vi "Unit Test.vi"() -> ()   [LabVIEW 2018]
uses:
  LWS SLA-070/Distro/Projects/12170 Luminar LWS Base/Source/PPLs/Oscilloscope.lvlibp/Oscilloscope.lvclass
  PicoScope 3000a.lvclass
  C:/Projects/LWS SLA-070/Distro/Projects/12170 Luminar LWS Base/Source/PPLs/Oscilloscope.lvlibp/Oscilloscope.lvclass
  PicoScope 3000a.lvclass/PicoScope 3000a.ctl
  LWS SLA-070/Distro/Projects/12170 Luminar LWS Base/Source/PPLs/Oscilloscope.lvlibp/Custom Controls/Analog Channels.ctl
  LWS SLA-070/Distro/Projects/12170 Luminar LWS Base/Source/PPLs/Oscilloscope.lvlibp/Custom Controls/Volts per Division.ctl
  LWS SLA-070/Distro/Projects/12170 Luminar LWS Base/Source/PPLs/Oscilloscope.lvlibp
  ps3000a.dll
panel:
  out "Handle":i16
  in  "TimePicoSeconds":i32
  in  "Interleave":i16
  in  "Cycles":i16
  in  "ETS_Mode":i32
  out "Oscilloscope out":refnum<class "Oscilloscope.lvclass">
  out "Multiple Waveform":waveform(dbl)[](graph)
  in  "Waveform":enum16{"Single", "Multiple"}(ring)
  in  "Secs/div":dbl
  out "SingleWaveform":waveform(dbl)(graph)
  in  "Acquire":bool
  in  "Set Scale":bool
  in  "Stop":bool
  out "error out":errorcluster
  in  "error in (no error)":errorcluster
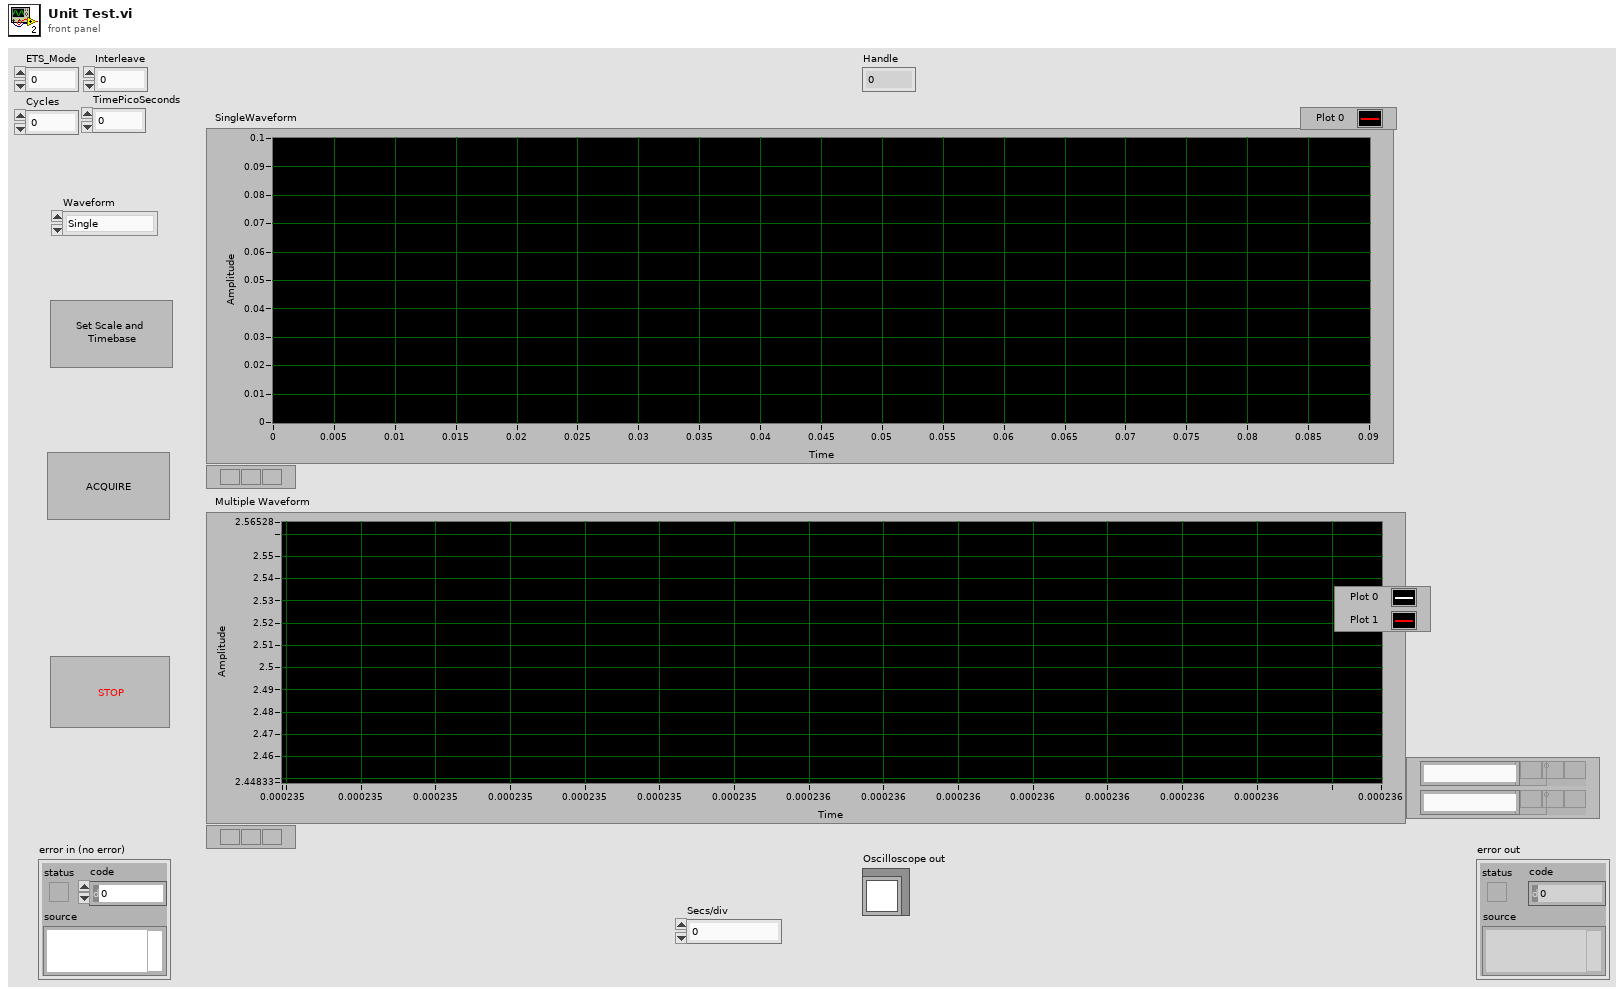
[diagram p1: front panel]
types:
  T1 = typedef "Oscilloscope.lvlibp/Analog Channels.ctl" = enum16{"1", "2", "3", "4", "5", "6", "7", "8", "9", "10", "11", "12", "13", "14", "15", "16"}
  T2 = typedef "Oscilloscope.lvlibp/Volts per Division.ctl" = cluster{"Analog Channels":T1, "V/div":dbl}[]
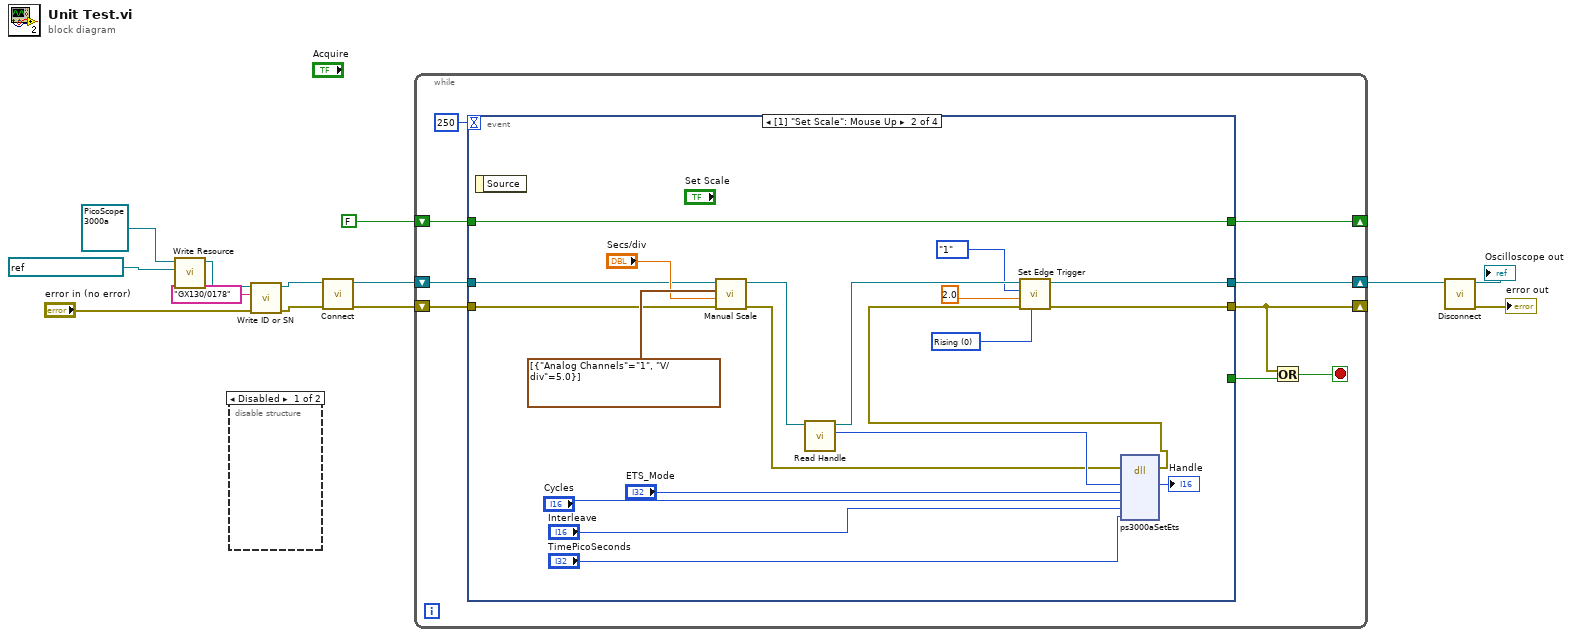
[diagram p0: block diagram]
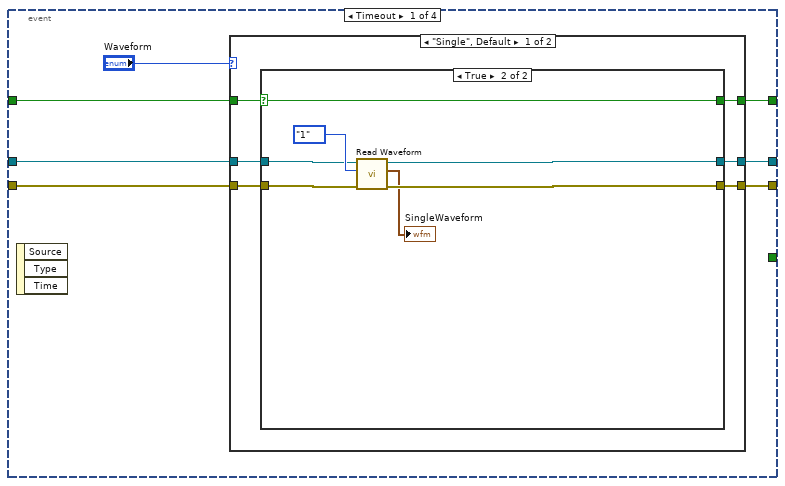
[diagram p3: hidden frame]
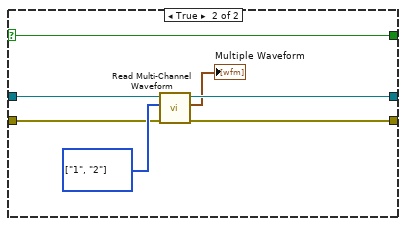
[diagram p6: hidden frame]
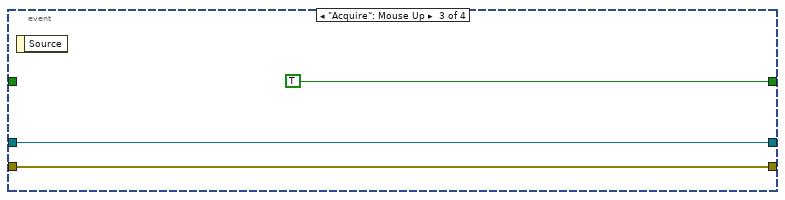
[diagram p7: hidden frame]
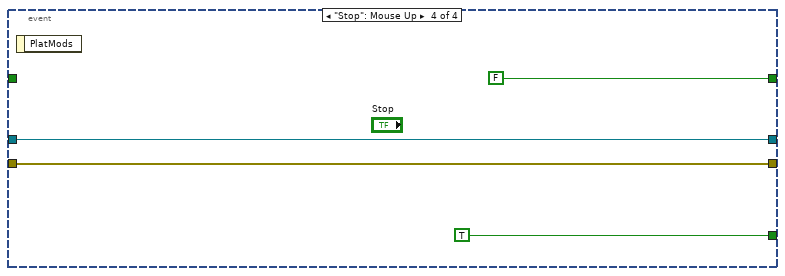
[diagram p8: hidden frame]
diagram:
  n1 = call "Write Resource.vi"("Resource"=refnum<visa-resource-name> "GX130/0178", "Oscilloscope in"=refnum<class "PicoScope 3000a.lvclass"> refnum ("PicoScope 3000a in")) -> ("Oscilloscope out"=w3:refnum<class "PicoScope 3000a.lvclass">)  [unwired: 8 in, 1 out]
  n2 = disable-structure shown="Disabled" {
    frame Disabled {
    }
    frame Enabled {
    }
  }
  n3 = call "Write ID or SN.vi"("error in (no error)"="error in (no error)", "ID or SN"="GX130/0178", "PicoScope 3000a in"=w3) -> ("error out"=w6:errorcluster, "PicoScope 3000a out"=w1:refnum<class "PicoScope 3000a.lvclass">)  [unwired: 7 in]
  n4 = call-dynamic "Connect.vi"("error in (no error)"=w6, "PicoScope 3000a in"=w1) -> ("error out"=w12:errorcluster, "PicoScope 3000a out"=w13:refnum<class "PicoScope 3000a.lvclass">)  [unwired: 8 in]
  n5 = while {
    shift-right: [w21] -> w10
    shift-left: w13 -> [w22]
    shift-right: [w15] -> _
    shift-left: w12 -> [w20]
    shift-right: [w18] -> _
    shift-left: FALSE -> [w19]
    stop <- w14 stop-if-true
    n6 = event shown="[1] \"Set Scale\": Mouse Up" {
      selector: _ -> [_ _ _ _]
      dyn-events: _ -> [_ _ _ _]
      timeout: 250 -> [_ _ _ _]
      tunnel: w22 -> [w27 w76 w84 w86]
      tunnel: [w26 w80 w84 w86] -> w21
      tunnel: w20 -> [w29 w75 w83 w85]
      tunnel: [w28 w79 w83 w85] -> w15
      tunnel: [_ _ _ TRUE] -> w16
      tunnel: w19 -> [w25 w81 _ _]
      tunnel: [w24 w81 TRUE FALSE] -> w18
      event Timeout {
        n7 = event-data() -> ()  [unwired: 1 in, 3 out]
        n8 = case shown="\"Single\", Default" "Waveform" {
          tunnel: w29 -> [w35 w46]
          tunnel: [w34 w47] -> w28
          tunnel: w27 -> [w33 w49]
          tunnel: [w32 w48] -> w26
          tunnel: w25 -> [w31 w50]
          tunnel: [w30 w51] -> w24
          frame "Single", Default {
            n9 = case shown="True" w31 {
              selector: w31 -> [w36 w40]
              tunnel: w35 -> [w37 w44]
              tunnel: [w37 w43] -> w34
              tunnel: w33 -> [w38 w42]
              tunnel: [w38 w41] -> w32
              tunnel: [w36 w40] -> w30
              frame False {
              }
              frame True {
                n10 = call-dynamic "Read Waveform.vi"("error in (no error)"=w44, "Channel"=Analog_Channels."1", "PicoScope 3000a in"=w42) -> ("error out"=w43:errorcluster, "Waveform"=→"SingleWaveform":waveform(dbl), "PicoScope 3000a out"=w41:refnum<class "PicoScope 3000a.lvclass">)  [unwired: 6 in]
              }
            }
          }
          frame "Multiple" {
            n11 = case shown="False" w50 {
              selector: w50 -> [w54 w61]
              tunnel: [w54 w61] -> w51
              tunnel: w49 -> [w53 w60]
              tunnel: [w53 w59] -> w48
              tunnel: [w52 w56] -> w47
              tunnel: w46 -> [w52 w57]
              frame False {
              }
              frame True {
                w58 = T1[] [enum."1", enum."2"] items=["1", "2", "3", "4", "5", "6", "7", "8", "9", "10", "11", "12", "13", "14", "15", "16"] ("Channels")
                n12 = call-dynamic "Read Multi-Channel Waveform.vi"("error in (no error)"=w57, "Channels"=w58, "PicoScope 3000a in"=w60) -> ("error out"=w56:errorcluster, "Waveform"=→"Multiple Waveform":waveform(dbl)[], "PicoScope 3000a out"=w59:refnum<class "PicoScope 3000a.lvclass">)  [unwired: 6 in]
              }
            }
          }
        }
      }
      event "Set Scale": Mouse Up {
        w62 = u16 0 items=["Rising", "Falling", "Either"] ("Trigger Slope (0: Rising)")
        n13 = event-data() -> ()  [unwired: 1 in, 1 out]
        n14 = call-dynamic "Manual Scale.vi"("error in (no error)"=w75, "Secs/div"="Secs/div", "V/div"=T2 [{"Analog Channels"=enum."1", "V/div"=5.0}], "PicoScope 3000a in"=w76) -> ("error out"=w68:errorcluster, "PicoScope 3000a out"=w66:refnum<class "PicoScope 3000a.lvclass">)  [unwired: 6 in]
        n15 = call "Read Handle.vi"("PicoScope 3000a in"=w66) -> ("Handle"=w74:i16, "PicoScope 3000a out"=w65:refnum<class "PicoScope 3000a.lvclass">)  [unwired: 8 in, 1 out]
        n16 = dll-call lib="ps3000a.dll" fn="ps3000aSetEts"(error in=w68, "Handle"=w74, "ETS_Mode"="ETS_Mode", "Cycles"="Cycles", "Interleave"="Interleave", "TimePicoSeconds"="TimePicoSeconds") -> (error out=w67:errorcluster, "Handle"=→"Handle":i16)  [unwired: 7 in, 1 out]
        n17 = call-dynamic "Set Edge Trigger.vi"("Trigger Slope (0: Rising)"=w62, "error in (no error)"=w67, "Trigger Level (0.0 V)"=2.0, "Analog Channel"=Analog_Channels."1", "PicoScope 3000a in"=w65) -> ("error out"=w79:errorcluster, "PicoScope 3000a out"=w80:refnum<class "PicoScope 3000a.lvclass">)  [unwired: 5 in]
      }
      event "Acquire": Mouse Up {
        n18 = event-data() -> ()  [unwired: 1 in, 1 out]
      }
      event "Stop": Mouse Up {
        n19 = event-data() -> ()  [unwired: 1 in, 1 out]
      }
    }
    n20 = Or(x=w15, y=w16) -> (x .or. y?=w14:bool)
  }
  n21 = call-dynamic "Disconnect.vi"("PicoScope 3000a in"=w10) -> ("error out"=→"error out":errorcluster, "PicoScope 3000a out"=→"Oscilloscope out":refnum<class "PicoScope 3000a.lvclass">)  [unwired: 9 in]
